vi "LD2018_ブロック崩し_BALL位置検出.vi"(1 "行/列数":i32, 2 "BALL座標":i32, 3 "オフセット":i32=3, 4 "幅/高さ":i32=49) -> (0 "位置":i32)   [LabVIEW 2017]
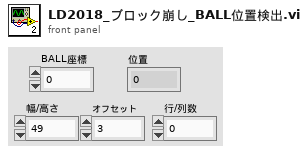
[diagram p1: front panel]
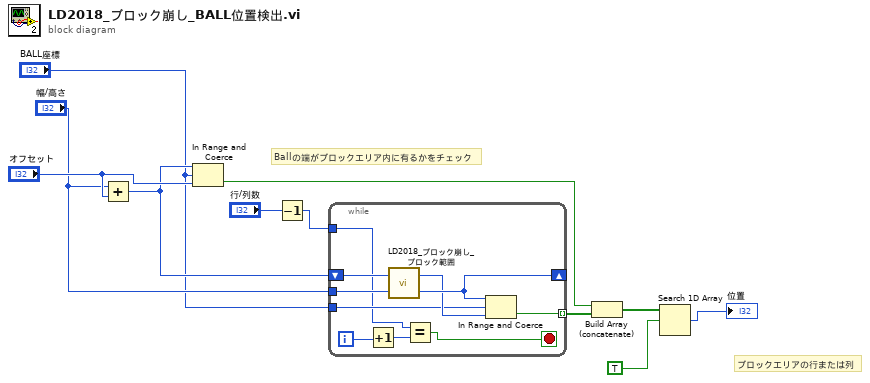
[diagram p0: block diagram]
diagram:
  # "ブロックエリアの行または列"
  # "Ballの端がブロックエリア内に有るかをチェック"
  n1 = Add(x="幅/高さ", y="オフセット") -> (x+y=w8:i32)
  n2 = In Range and Coerce(upper limit=w8, x="BALL座標", lower limit="オフセット") -> (In Range?=w7:bool)  [unwired: 1 out]
  n3 = Decrement(x="行/列数") -> (x-1=w1:i32)
  n4 = while "Forループ" {
    shift-right: [w20] -> _
    shift-left: w8 -> [w21]
    tunnel: [w18] -> w6 mode=indexing
    tunnel: "幅/高さ" -> [w17]
    tunnel: "BALL座標" -> [w16]
    tunnel: w1 -> [w13]
    i -> [w15]
    stop <- w12 stop-if-true
    n5 = Increment(x=w15) -> (x+1=w14:i32)
    n6 = call "LD2018_ブロック崩し_ブロック範囲.vi"("長さ/幅"=w17, "直前エリア位置"=w21) -> ("最大値"=w20:i32, "最小値"=w19:i32)
    n7 = Equal?(x=w13, y=w14) -> (x = y?=w12:bool)
    n8 = In Range and Coerce(upper limit=w20, x=w16, lower limit=w19) -> (In Range?=w18:bool)  [unwired: 1 out]
  }
  n9 = Build Array (concatenate)(w7, w6) -> (w5:bool[])
  n10 = Search 1D Array(1D array=w5, element=TRUE ("要素")) -> (index of element=→"位置":i32)  [unwired: 1 in]
